vi "Parse-broadcast-data-status.vi"(8 "error in (no error)":errorcluster, 10 "Multiple device identification XML string":string="<LecList>\n  <Lec name='EC_Alpha' ip='192.168.42.30' mac='address' />\n  <Lec name='EC_Beta' ip='192.168.42.31' mac='addressB' />\n</LecList>") -> (0 "error out":errorcluster, 2 "Status information":T1)   [LabVIEW 2013, in "SLMControl.lvlib" / "SM1000.lvclass"]
uses:
  SM1000.lvclass
  Status-information.ctl
  <vilib>/xml/Load XML String.vi
  <vilib>/xml/Close Reference(Node).vi
  <vilib>/xml/NI_XML.lvlib
  <resource>/objmgr/DOMUserDefRef.rc
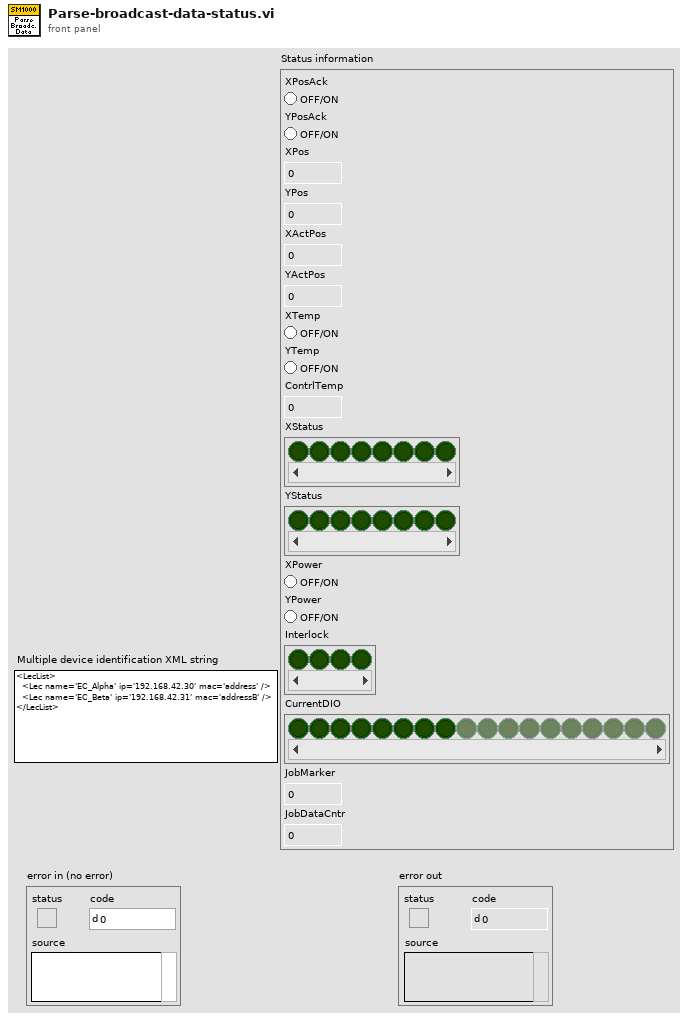
[diagram p1: front panel]
types:
  T1 = typedef "SLMControl.lvlib/SM1000.lvclass/Status-information.ctl" = cluster{"XPosAck":bool, "YPosAck":bool, "XPos":i16, "YPos":i16, "XActPos":i16, "YActPos":i16, "XTemp":bool, "YTemp":bool, "ContrlTemp":i16, "XStatus":bool[], "YStatus":bool[], "XPower":bool, "YPower":bool, "Interlock":bool[], "CurrentDIO":bool[], "JobMarker":u16, "JobDataCntr":u32}
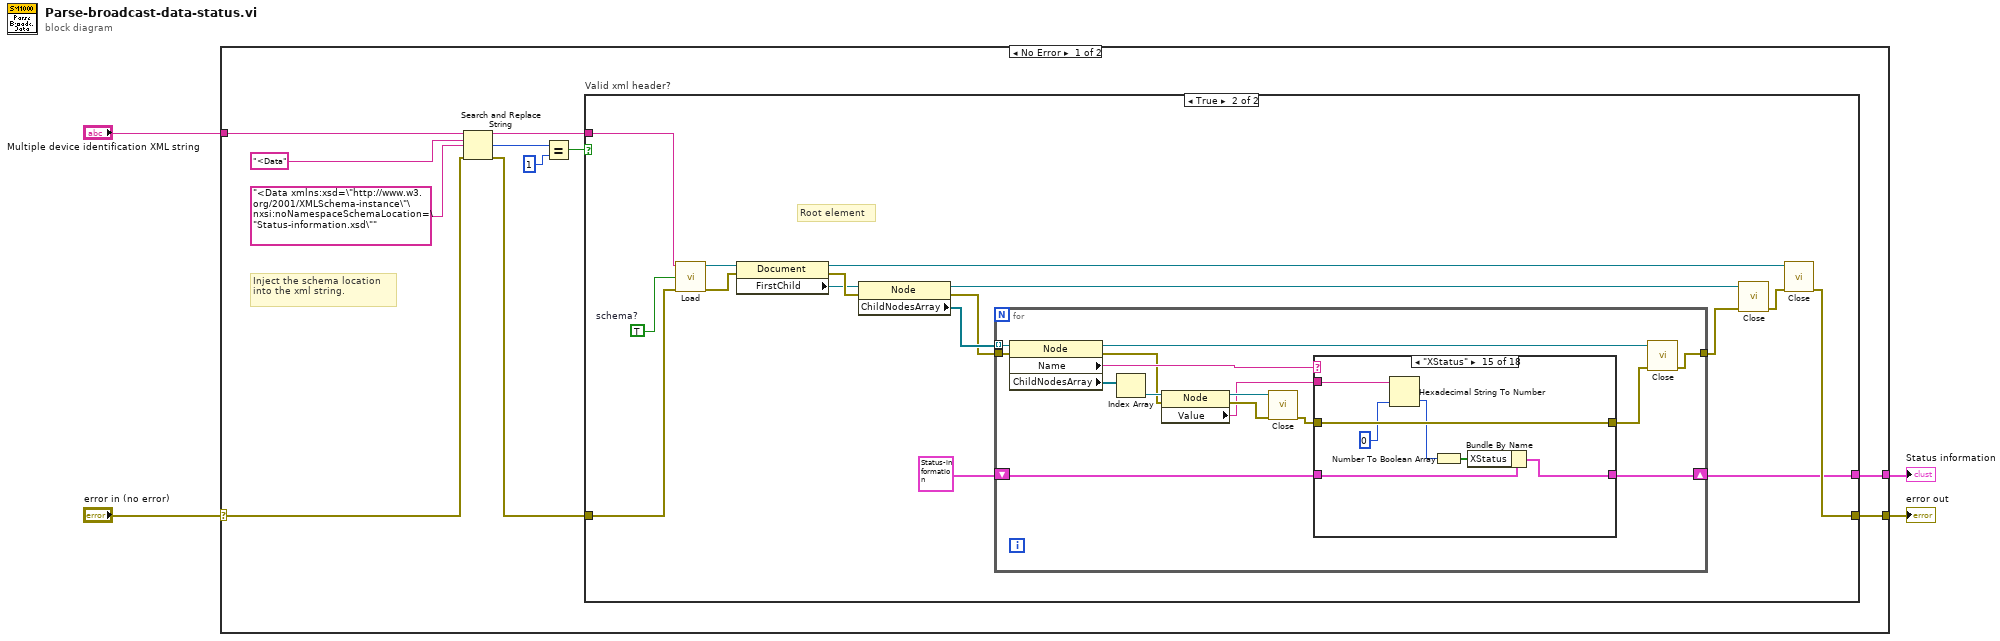
[diagram p0: block diagram]
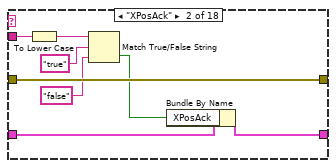
[diagram p4: hidden frame]
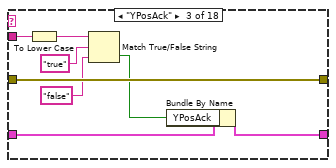
[diagram p5: hidden frame]
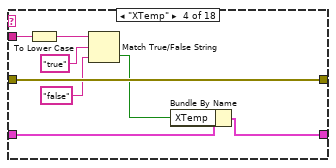
[diagram p6: hidden frame]
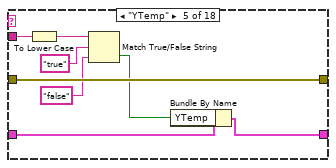
[diagram p7: hidden frame]
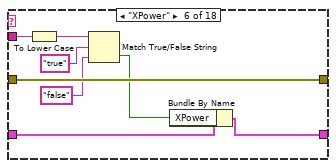
[diagram p8: hidden frame]
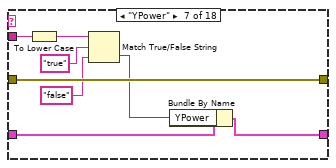
[diagram p9: hidden frame]
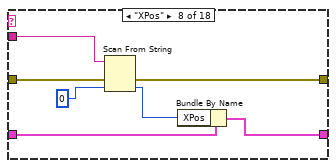
[diagram p10: hidden frame]
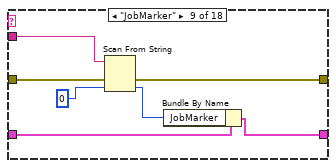
[diagram p11: hidden frame]
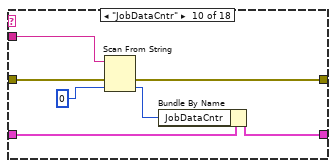
[diagram p12: hidden frame]
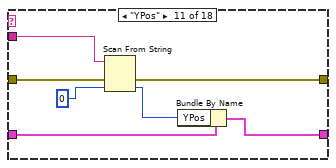
[diagram p13: hidden frame]
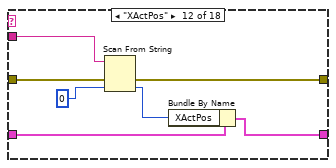
[diagram p14: hidden frame]
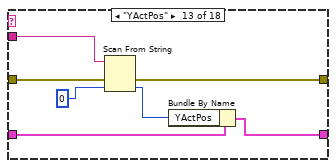
[diagram p15: hidden frame]
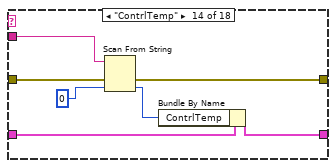
[diagram p16: hidden frame]
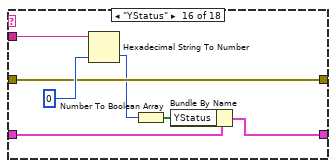
[diagram p17: hidden frame]
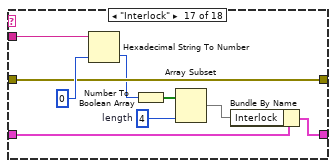
[diagram p18: hidden frame]
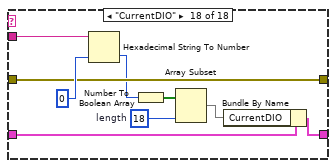
[diagram p19: hidden frame]
diagram:
  n1 = case shown="No Error" "error in (no error)" {
    selector: "error in (no error)" -> [w12 w179]
    tunnel: [w7 w179] -> w3
    tunnel: "Multiple device identification XML string" -> [w15 _]
    tunnel: [w5 _] -> w1
    frame No Error {
      # "Inject the schema location\ninto the xml string."
      n2 = Search and Replace String(input string=w15, search string="<Data", replace string="<Data xmlns:xsd=\"http://www.w3.org/2001/XMLSchema-instance\"\nxsi:noNamespaceSchemaLocation=\"Status-information.xsd\"", error in=w12) -> (result string=w8:string, number of replacements=w11:i32, error out=w6:errorcluster)  [unwired: 4 in, 1 out]
      n3 = Equal?(x=w11, y=1) -> (x = y?=w9:bool)
      n4 = case "Valid xml header?" shown="True" w9 {
        tunnel: w8 -> [_ w19]
        tunnel: [w16 w28] -> w7
        tunnel: w6 -> [w16 w29]
        tunnel: [_ w17] -> w5
        frame False {
        }
        frame True {
          w32 = TRUE  # schema?
          # "Root element"
          n5 = call-poly <vilib>:"Load.vi"("XML string"=w19, "process schema (False)"=w32, "error in (no error)"=w29) -> ("DOM document out"=w31:refnum<k20>, "error out"=w30:errorcluster)  [unwired: 10 in, 1 out]
          n6 = property class="Document"(reference=w31, error in=w30) -> (reference out=w21:refnum<k20>, error out=w23:errorcluster, "FirstChild"=w20:refnum<k20>)
          n7 = property class="Node"(reference=w20, error in=w23) -> (reference out=w22:refnum<k20>, error out=w24:errorcluster, "ChildNodesArray"=w25:refnum<k20>[])
          n8 = for {
            tunnel: w25 -> [w47] mode=indexing
            tunnel: w24 -> [w46]
            tunnel: [w43] -> w27
            shift-right: [w40] -> w17
            shift-left: T1 {"XPosAck"=FALSE, "YPosAck"=FALSE, "XPos"=0, "YPos"=0, "XActPos"=0, "YActPos"=0, "XTemp"=FALSE, "YTemp"=FALSE, "ContrlTemp"=0, "XStatus"=[FALSE, FALSE, FALSE, FALSE, FALSE, FALSE, FALSE, FALSE], "YStatus"=[FALSE, FALSE, FALSE, FALSE, FALSE, FALSE, FALSE, FALSE], "XPower"=FALSE, "YPower"=FALSE, "Interlock"=[FALSE, FALSE, FALSE, FALSE], "CurrentDIO"=[FALSE, FALSE, FALSE, FALSE, FALSE, FALSE, FALSE, FALSE, FALSE, FALSE, FALSE, FALSE, FALSE, FALSE, FALSE, FALSE, FALSE, FALSE], "JobMarker"=0, "JobDataCntr"=0} ("Status information") -> [w41]
            n9 = property class="Node"(reference=w47, error in=w46) -> (reference out=w45:refnum<k20>, error out=w37:errorcluster, "Name"=w42:string, "ChildNodesArray"=w39:refnum<k20>[])
            n10 = Index Array(array=w39) -> (element=w38:refnum<k20>)  [unwired: 1 in]
            n11 = property class="Node"(reference=w38, error in=w37) -> (reference out=w34:refnum<k20>, error out=w36:errorcluster, "Value"=w33:string)
            n12 = call-poly <vilib>:"Close.vi"("error in (no error)"=w36, "node"=w34) -> ("error out"=w35:errorcluster)  [unwired: 7 in]
            n13 = case shown="\"XStatus\"" w42 {
              tunnel: w35 -> [w49 w54 w62 w70 w78 w86 w94 w102 w109 w116 w123 w130 w137 w144 w149 w155 w162 w171]
              tunnel: [w49 w54 w62 w70 w78 w86 w94 w98 w105 w112 w119 w126 w133 w140 w149 w155 w162 w171] -> w44
              tunnel: w41 -> [w48 w57 w65 w73 w81 w89 w97 w104 w111 w118 w125 w132 w139 w146 w153 w160 w169 w178]
              tunnel: w33 -> [_ w55 w63 w71 w79 w87 w95 w101 w108 w115 w122 w129 w136 w143 w151 w156 w163 w172]
              tunnel: [w48 w56 w64 w72 w80 w88 w96 w103 w110 w117 w124 w131 w138 w145 w152 w159 w168 w177] -> w40
              frame Default {
              }
              frame "XPosAck" {
                n14 = To Lower Case(string=w55) -> (all lower case string=w53:string)
                n15 = Match True/False String(2:"false", 3:"true", 4:w53) -> (0:w50:bool)  [unwired: 1 out]
                n16 = Bundle By Name(cluster=w57, "XPosAck"=w50) -> (w56:T1)
              }
              frame "YPosAck" {
                n17 = To Lower Case(string=w63) -> (all lower case string=w61:string)
                n18 = Match True/False String(2:"false", 3:"true", 4:w61) -> (0:w58:bool)  [unwired: 1 out]
                n19 = Bundle By Name(cluster=w65, "YPosAck"=w58) -> (w64:T1)
              }
              frame "XTemp" {
                n20 = To Lower Case(string=w71) -> (all lower case string=w69:string)
                n21 = Match True/False String(2:"false", 3:"true", 4:w69) -> (0:w66:bool)  [unwired: 1 out]
                n22 = Bundle By Name(cluster=w73, "XTemp"=w66) -> (w72:T1)
              }
              frame "YTemp" {
                n23 = To Lower Case(string=w79) -> (all lower case string=w77:string)
                n24 = Match True/False String(2:"false", 3:"true", 4:w77) -> (0:w74:bool)  [unwired: 1 out]
                n25 = Bundle By Name(cluster=w81, "YTemp"=w74) -> (w80:T1)
              }
              frame "XPower" {
                n26 = To Lower Case(string=w87) -> (all lower case string=w85:string)
                n27 = Match True/False String(2:"false", 3:"true", 4:w85) -> (0:w82:bool)  [unwired: 1 out]
                n28 = Bundle By Name(cluster=w89, "XPower"=w82) -> (w88:T1)
              }
              frame "YPower" {
                n29 = To Lower Case(string=w95) -> (all lower case string=w93:string)
                n30 = Match True/False String(2:"false", 3:"true", 4:w93) -> (0:w90:bool)  [unwired: 1 out]
                n31 = Bundle By Name(cluster=w97, "YPower"=w90) -> (w96:T1)
              }
              frame "XPos" {
                n32 = Scan From String(input string=w101, error in=w102, default 1=i16 0) -> (error out=w98:errorcluster, output 1=w99:i16)  [unwired: 2 in, 2 out]
                n33 = Bundle By Name(cluster=w104, "XPos"=w99) -> (w103:T1)
              }
              frame "JobMarker" {
                n34 = Scan From String(input string=w108, error in=w109, default 1=u16 0) -> (error out=w105:errorcluster, output 1=w106:u16)  [unwired: 2 in, 2 out]
                n35 = Bundle By Name(cluster=w111, "JobMarker"=w106) -> (w110:T1)
              }
              frame "JobDataCntr" {
                n36 = Scan From String(input string=w115, error in=w116, default 1=u32 0) -> (error out=w112:errorcluster, output 1=w113:u32)  [unwired: 2 in, 2 out]
                n37 = Bundle By Name(cluster=w118, "JobDataCntr"=w113) -> (w117:T1)
              }
              frame "YPos" {
                n38 = Scan From String(input string=w122, error in=w123, default 1=i16 0) -> (error out=w119:errorcluster, output 1=w120:i16)  [unwired: 2 in, 2 out]
                n39 = Bundle By Name(cluster=w125, "YPos"=w120) -> (w124:T1)
              }
              frame "XActPos" {
                n40 = Scan From String(input string=w129, error in=w130, default 1=i16 0) -> (error out=w126:errorcluster, output 1=w127:i16)  [unwired: 2 in, 2 out]
                n41 = Bundle By Name(cluster=w132, "XActPos"=w127) -> (w131:T1)
              }
              frame "YActPos" {
                n42 = Scan From String(input string=w136, error in=w137, default 1=i16 0) -> (error out=w133:errorcluster, output 1=w134:i16)  [unwired: 2 in, 2 out]
                n43 = Bundle By Name(cluster=w139, "YActPos"=w134) -> (w138:T1)
              }
              frame "ContrlTemp" {
                n44 = Scan From String(input string=w143, error in=w144, default 1=i16 0) -> (error out=w140:errorcluster, output 1=w141:i16)  [unwired: 2 in, 2 out]
                n45 = Bundle By Name(cluster=w146, "ContrlTemp"=w141) -> (w145:T1)
              }
              frame "XStatus" {
                n46 = Hexadecimal String To Number(string=w151, default (0uL)=u8 0) -> (number=w147:u8)  [unwired: 1 in, 1 out]
                n47 = Number To Boolean Array(number=w147) -> (Boolean array=w150:bool[])
                n48 = Bundle By Name(cluster=w153, "XStatus"=w150) -> (w152:T1)
              }
              frame "YStatus" {
                n49 = Hexadecimal String To Number(string=w156, default (0uL)=u8 0) -> (number=w154:u8)  [unwired: 1 in, 1 out]
                n50 = Number To Boolean Array(number=w154) -> (Boolean array=w158:bool[])
                n51 = Bundle By Name(cluster=w160, "YStatus"=w158) -> (w159:T1)
              }
              frame "Interlock" {
                w165 = 4  # length
                n52 = Hexadecimal String To Number(string=w163, default (0uL)=u32 0) -> (number=w161:u32)  [unwired: 1 in, 1 out]
                n53 = Number To Boolean Array(number=w161) -> (Boolean array=w166:bool[])
                n54 = Array Subset(array=w166, length=w165) -> (w167:bool[])  [unwired: 1 in]
                n55 = Bundle By Name(cluster=w169, "Interlock"=w167) -> (w168:T1)
              }
              frame "CurrentDIO" {
                w174 = 18  # length
                n56 = Hexadecimal String To Number(string=w172, default (0uL)=u32 0) -> (number=w170:u32)  [unwired: 1 in, 1 out]
                n57 = Number To Boolean Array(number=w170) -> (Boolean array=w175:bool[])
                n58 = Array Subset(array=w175, length=w174) -> (w176:bool[])  [unwired: 1 in]
                n59 = Bundle By Name(cluster=w178, "CurrentDIO"=w176) -> (w177:T1)
              }
            }
            n60 = call-poly <vilib>:"Close.vi"("error in (no error)"=w44, "node"=w45) -> ("error out"=w43:errorcluster)  [unwired: 7 in]
          }
          n61 = call-poly <vilib>:"Close.vi"("error in (no error)"=w27, "node"=w22) -> ("error out"=w26:errorcluster)  [unwired: 7 in]
          n62 = call-poly <vilib>:"Close.vi"("error in (no error)"=w26, "node"=w21) -> ("error out"=w28:errorcluster)  [unwired: 7 in]
        }
      }
    }
    frame Error {
    }
  }
  "error out" <- w3
  "Status information" <- w1
